vi "GV FIFOOUTgate.vi"() -> ()   [LabVIEW 2017]
panel:
  out "FIFOOUTgate":bool
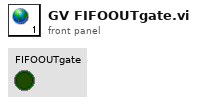
[diagram p1: front panel]
diagram:
